vi "CSM - Global Log Event Monitoring Loop.vi"() -> ()   [LabVIEW 2017, in "CSM-QuickDrops.lvlib"]
doc: "Creates a global log event monitoring loop, which is used for querying and monitoring messages in the global log queue.\n\n<b>Reference Example</b>: Any examples in `[CSM-Example]\\4. Advance Examples\\4. Global Log Filter Example\\`."
uses:
  CSM-QuickDrops.lvlib
  _Support/Typedef/_CSM_GlobalLog_MSG.ctl
  _Support/Typedef/_CSM_Response Source Message.ctl
  _Support/Typedef/_CSM_GlobalLog_MSG_TYPE.ctl
  Utility/Periodic String Filter Setting.ctl
  Communicable State Machine.lvlib
  _Shared/CSM Shared.lvlib
panel:
  out "log handling Speed(#/s)":dbl
  in  "Stop":bool
  out "State History":string
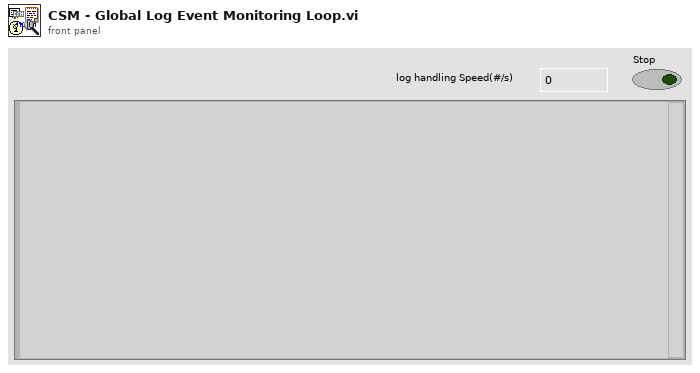
[diagram p1: front panel]
types:
  T1 = typedef "Communicable State Machine.lvlib/_CSM_GlobalLog_MSG.ctl" = cluster{"Name (\"\" to Use UUID)":string, "Current State":string, "Arguments":string, "Source Message":T2, "Source Module":string, "Complete(T)/Start(F)":bool, "LogType":T3, "Time Stamp":timestamp}
  T2 = typedef "Communicable State Machine.lvlib/_CSM_Response Source Message.ctl" = cluster{"‘State":string, "’Arguments":string, "’Error":errorcluster}
  T3 = typedef "Communicable State Machine.lvlib/_CSM_GlobalLog_MSG_TYPE.ctl" = enum16{"User Log", "State Change", "Status", "Interrupt", "Register", "Unregister", "Error Log", "Module Created", "Module Destroyed", "Async Message", "No-Rep Async Message", "Sync Message"}
  T4 = typedef "Communicable State Machine.lvlib/Periodic String Filter Setting.ctl" = cluster{"threashold(#/s)":dbl, "Check Peroid(s)":dbl}
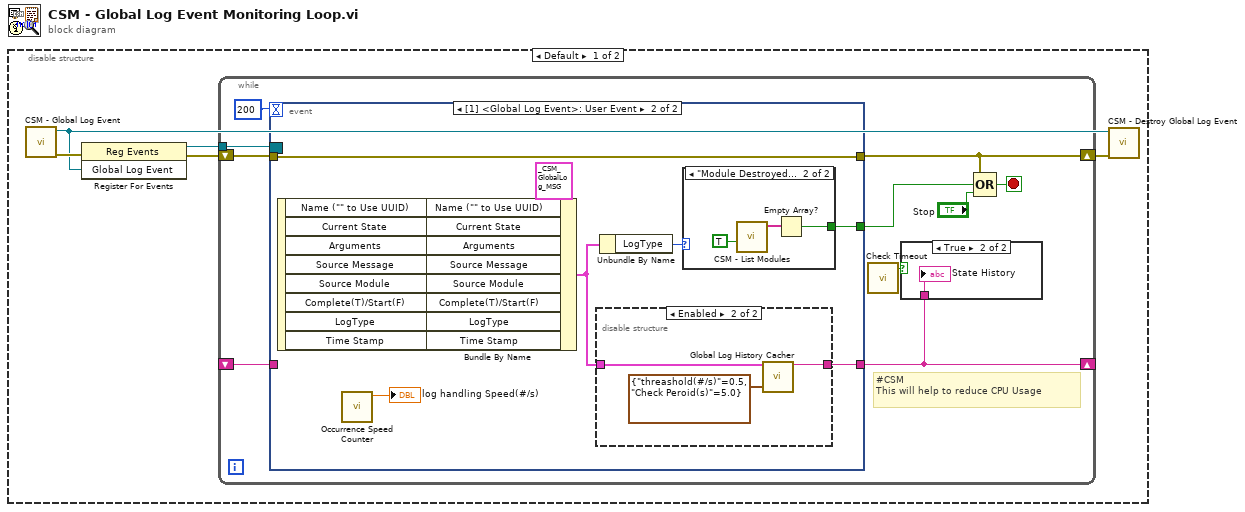
[diagram p0: block diagram]
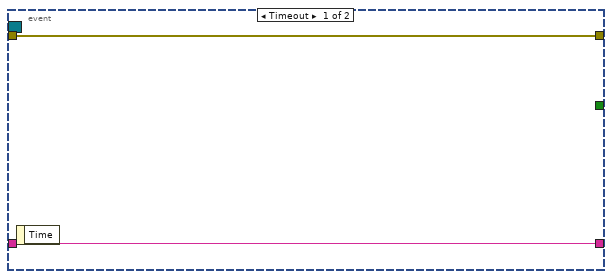
[diagram p3: hidden frame]
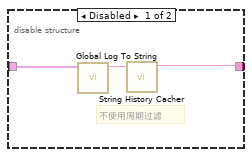
[diagram p4: hidden frame]
diagram:
  n1 = disable-structure shown="Default" {
    frame condition #0 (active) {
      n2 = call "CSM - Global Log Event.vi"() -> ("error out"=w3:errorcluster, "Global Log Event"=w1:refnum<user-event>)  [unwired: 10 in]
      n3 = register-events(error in=w3, w1) -> (reference out=w4:refnum<event-registration>, error out=w5:errorcluster)  [unwired: 1 in]
      n4 = while {
        tunnel: w4 -> [w15]
        shift-right: [w12] -> w2
        shift-left: w5 -> [w14]
        shift-right: [w9] -> _
        shift-left: _ -> [w8]
        stop <- w13 stop-if-true
        # "#CSM\nThis will help to reduce CPU Usage"
        n5 = event shown="[1] <Global Log Event>: User Event" {
          selector: w15 -> [_ _]
          dyn-events: _ -> [_ _]
          timeout: 200 -> [_ _]
          tunnel: w14 -> [w18 w33]
          tunnel: [w18 w33] -> w12
          tunnel: [_ w23] -> w11
          tunnel: [w17 w21] -> w9
          tunnel: w8 -> [w17 _]
          event Timeout {
            n6 = event-data() -> ()  [unwired: 1 in, 1 out]
          }
          event User Event {
            n7 = event-data() -> ("Name (\"\" to Use UUID)"=w32:string, "Current State"=w31:string, "Arguments"=w30:string, "Source Message"=w29:T2, "Source Module"=w28:string, "Complete(T)/Start(F)"=w27:bool, "LogType"=w26:T3, "Time Stamp"=w22:timestamp)  [unwired: 1 in]
            n8 = call "Occurrence Speed Counter.vi"() -> ("Speed (#/s)"=→"log handling Speed(#/s)":dbl)  [unwired: 9 in, 2 out]
            n9 = Bundle By Name(cluster=T1 {"Name (\"\" to Use UUID)"="", "Current State"="", "Arguments"="", "Source Message"={"‘State"="", "’Arguments"="", "’Error"={"status"=FALSE, "code"=0, "source"=""}}, "Source Module"="", "Complete(T)/Start(F)"=FALSE, "LogType"=enum."State Change", "Time Stamp"=timestamp(0 s since 1904-01-01)} ("Cross CSM Data"), "Name (\"\" to Use UUID)"=w32, "Current State"=w31, "Arguments"=w30, "Source Message"=w29, "Source Module"=w28, "Complete(T)/Start(F)"=w27, "LogType"=w26, "Time Stamp"=w22) -> (w20:T1)
            n10 = disable-structure shown="Enabled" {
              disable-tunnel: w20 -> [w36 w37]
              disable-tunnel: [w34 w39] -> w21
              frame Disabled {
                # "不使用周期过滤"
                n11 = call "Global Log To String.vi"("Log"=w36) -> ("Log String"=w35:string)  [unwired: 9 in]
                n12 = call "String History Cacher.vi"("String"=w35) -> ("String Cache"=w34:string)  [unwired: 10 in]
              }
              frame Enabled {
                n13 = call "Global Log History Cacher.vi"("Global Log Data"=w37, "Settings"=T4 {"threashold(#/s)"=0.5, "Check Peroid(s)"=5.0}) -> ("String Cache"=w39:string)  [unwired: 13 in]
              }
            }
            n14 = Unbundle By Name(w20) -> ("LogType"=w24:T3)
            n15 = case shown="\"Module Destroyed\"" w24 {
              tunnel: [_ w40] -> w23
              frame "User Log", Default {
              }
              frame "Module Destroyed" {
                n16 = call "CSM - List Modules.vi"("With Nodes? (F)"=TRUE ("All?")) -> ("Module Names"=w42:string[])  [unwired: 9 in, 1 out]
                n17 = Empty Array?(array=w42) -> (empty?=w40:bool)
              }
            }
          }
        }
        n18 = call "Check Timeout.vi"() -> ("Timeout"=w7:bool)  [unwired: 8 in]
        n19 = case shown="True" w7 {
          tunnel: w9 -> [_ w16]
          frame False {
          }
          frame True {
            "State History" <- w16
          }
        }
        n20 = Compound Arithmetic op=OR(w12, w11, "Stop") -> (w13:bool)
      }
      n21 = call "CSM - Destroy Global Log Event.vi"("Error In"=w2, "CSM Global Log Event"=w1) -> ()  [unwired: 9 in, 1 out]
    }
    frame condition #1 {
    }
  }
